vi "Queue Image (MMF) (SubVI).vi"(4 "TimeStamp":u64, 6 "Frame Number":u64, 8 "Experiment Mode":T1=enum."Replay", 10 "Image Size":T5={"Height"=512, "Width"=512}, 11 "Data Bundle":T2) -> ()   [LabVIEW 2020]
uses:
  Controls (HOST)/Image Size.ctl
  Controls (HOST)/REF.ctl
  Controls (HOST)/Image Queue Bundle.ctl
  Controls (HOST)/Data to Disk Bundle.ctl
  Controls (HOST)/File Name Prefix.ctl
  Controls (HOST)/FPGA REF (MWT).ctl
  Controls (HOST)/Experiment Mode.ctl
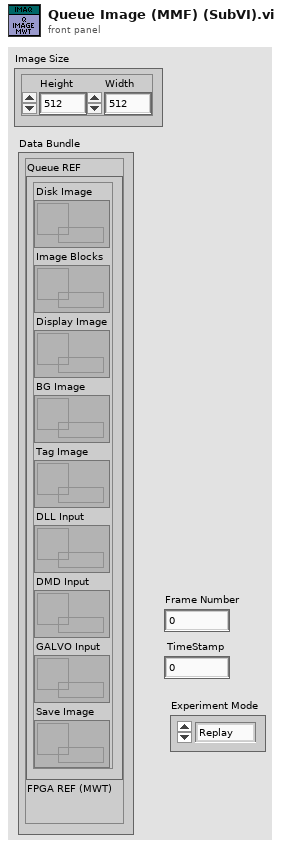
[diagram p1: front panel]
types:
  T1 = typedef "Experiment Mode.ctl" = enum16{"Live", "Replay"}
  T2 = typedef "REF.ctl" = cluster{"Queue REF":T3, "FPGA REF (MWT)":T4}
  T3 = typedef "Image Queue Bundle.ctl" = cluster{"Disk Image":refnum<queue>, "Image Blocks":refnum<queue>, "Display Image":refnum<queue>, "BG Image":refnum<queue>, "Tag Image":refnum<queue>, "DLL Input":refnum<queue>, "DMD Input":refnum<queue>, "GALVO Input":refnum<queue>, "Save Image":refnum<queue>}
  T4 = typedef "FPGA REF (MWT).ctl" = refnum<k20>
  T5 = typedef "Image Size.ctl" = cluster{"Height":u16, "Width":u16}
  T6 = typedef "Data to Disk Bundle.ctl" = cluster{"Frame Number":u64, "Time Stamp (us)":u64, "Image Data":u64[], "Contour":u32[], "Raw Image REF":refnum<data-value>, "Block Image REF":refnum<data-value>, "Block Box":u64[], "SPINE":u32[], "HT Angle":u64[], "Block Position":u64[], "SPINE Count":u32[], "Contour Count":u32[], "SPINE DIR":u8[]}
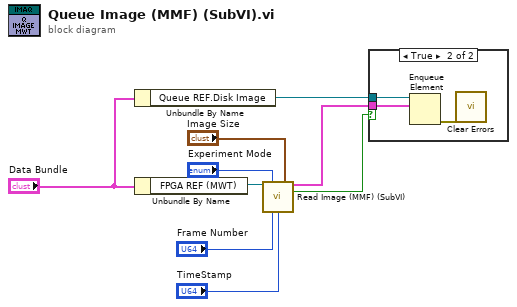
[diagram p0: block diagram]
diagram:
  n1 = Unbundle By Name("Data Bundle") -> ("Queue REF.Disk Image"=w7:refnum<queue>)
  n2 = Unbundle By Name("Data Bundle") -> ("FPGA REF (MWT)"=w9:T4)
  n3 = call "Read Image (MMF) (SubVI).vi"("FPGA REF (MWT) IN"=w9, "Experiment Mode"="Experiment Mode", "Image Size"="Image Size", "Frame Number"="Frame Number", "TimeStamp"="TimeStamp") -> ("Image Data"=w2:T6, "Data Valid?"=w1:bool)  [unwired: 9 in]
  n4 = case shown="True" w1 {
    tunnel: w7 -> [_ w12]
    tunnel: w2 -> [_ w11]
    frame False {
    }
    frame True {
      n5 = Enqueue Element(queue=w12, element=w11) -> (error out=w10:errorcluster)  [unwired: 2 in, 2 out]
      n6 = call <vilib>:"Clear Errors.vi"("error in (no error)"=w10) -> ()  [unwired: 5 in, 2 out]
    }
  }
